vi "Resample Wfm Linear Open Interval.vi"(10 "Sample Rate":dbl, 11 "Original Waveforms":waveform(dbl)[](array[waveform])) -> (2 "Resampled Waveform":waveform(dbl)[](array[waveform]), 3 "Waveform Names":string[](array[string]))   [LabVIEW 2021]
uses:
  <vilib>/express/express shared/transition.llb/Dynamic To Waveform Array.vi
  <vilib>/express/express signal manip/GetorSetDDTAttributes/Set DDT Attributes/SetT0.vi
  <vilib>/express/express shared/transition.llb/Waveform Array To Dynamic.vi
  <vilib>/express/express signal manip/GetorSetDDTAttributes/Get DDT Attributes/Get DDT Properties.xnode
  <vilib>/express/express signal manip/GetorSetDDTAttributes/Set DDT Attributes/Set DDT Properties.xnode
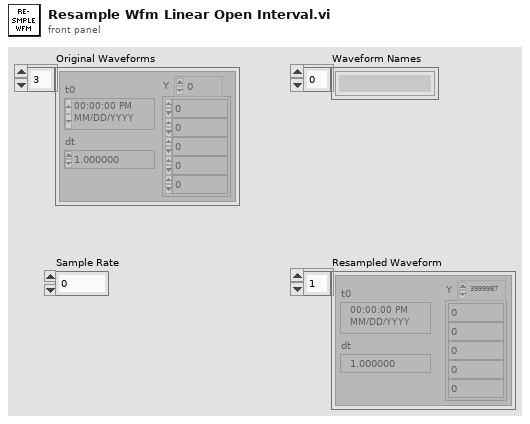
[diagram p1: front panel]
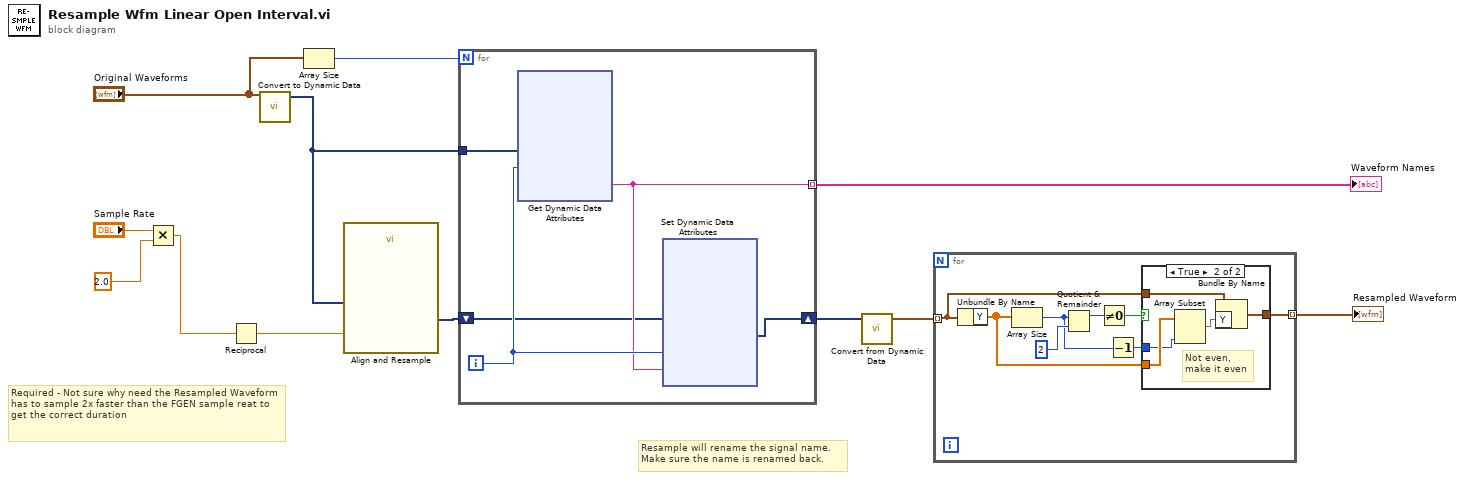
[diagram p0: block diagram]
diagram:
  # "Required - Not sure why need the Resampled Waveform has to sample 2x faster than the FGEN sample reat to get the correct duration"
  # "Resample will rename the signal name.\nMake sure the name is renamed back."
  n1 = Multiply(x="Sample Rate", y=2.0) -> (x*y=w4:dbl)
  n2 = Reciprocal(x=w4) -> (1/x=w6:dbl)
  n3 = call "Convert to Dynamic Data"("Array of Waveforms"="Original Waveforms") -> ("Dynamic Data Type"=w12:dynamicdata)  [unwired: 3 in]
  n4 = Array Size(array="Original Waveforms") -> (size(s)=w8:i32)
  n5 = call "Align and Resample"("dt"=w6, "Signals"=w12) -> ("Resampled Signals"=w10:dynamicdata)  [unwired: 7 in, 2 out]
  n6 = for {
    N: w8 -> [_]
    tunnel: [w16] -> w9 mode=indexing
    shift-right: [w15] -> w11
    shift-left: w10 -> [w14]
    tunnel: w12 -> [w13]
    i -> [w17]
    n7 = xnode "Get Dynamic Data Attributes"("Signals In"=w13, "Signal Index"=w17) -> ("Signal Name"=w16:string)  [unwired: 1 in, 2 out]
    n8 = xnode "Set Dynamic Data Attributes"("Signals In"=w14, "Signal Index"=w17, "Signal Name"=w16) -> ("Signals Out"=w15:dynamicdata)  [unwired: 1 in, 1 out]
  }
  "Waveform Names" <- w9
  n9 = call "Convert from Dynamic Data"("Dynamic Data Type"=w11) -> ("Array of Waveform"=w2:waveform(dbl)[])  [unwired: 3 in]
  n10 = for {
    tunnel: w2 -> [w44] mode=indexing
    tunnel: [w40] -> w1 mode=indexing
    n11 = Unbundle By Name(w44) -> ("Y"=w43:dbl[])
    n12 = Array Size(array=w43) -> (size(s)=w42:i32)
    n13 = Quotient & Remainder(x=w42, y=2) -> (x-y*floor(x/y)=w46:i32)  [unwired: 1 out]
    n14 = Not Equal To 0?(x=w46) -> (x != 0?=w45:bool)
    n15 = Decrement(x=w42) -> (x-1=w41:i32)
    n16 = case shown="True" w45 {
      tunnel: w44 -> [w48 w53]
      tunnel: w43 -> [_ w52]
      tunnel: w41 -> [_ w51]
      tunnel: [w48 w49] -> w40
      frame False {
      }
      frame True {
        # "Not even,\nmake it even"
        n17 = Array Subset(array=w52, length=w51) -> (w50:dbl[])  [unwired: 1 in]
        n18 = Bundle By Name(cluster=w53, "Y"=w50) -> (w49:waveform(dbl))
      }
    }
  }
  "Resampled Waveform" <- w1
